vi "accelTest.vi"(0 "Communication in":refnum<class "Communication.lvclass">, 1 "Game":refnum<class "Game.lvclass">, 2 "id":i32, 3 "V_accel":dbl, 4 "V_deaccel":dbl, 5 "error in (no error)":errorcluster, 6 "replace active":bool, 7 "Samples":dbl, 8 "Start":bool=TRUE) -> (14 "Communication out":refnum<class "Communication.lvclass">, 15 "Replace":bool, 16 "Game out":refnum<class "Game.lvclass">, 19 "error out":errorcluster)   [LabVIEW 2021, in "Communication.lvclass"]
uses:
  Communication.lvclass
  Game_class/Game.lvclass
  Controls/RobotModel.ctl
  Utilities_class/Utilities.lvclass
  Game_class/Game.lvclass/Game.ctl
  Team_class/Team.lvclass/Team.ctl
  Robot_class/Robot.lvclass/Robot.ctl
  Object_class/Object.lvclass/Object.ctl
  Robot_class/Read est_v_tang.vi
  Robot_class/Write v_tang.vi
  Robot_class/Write v_norm.vi
  Robot_class/Write v_ang.vi
  Object_class/Read x.vi
  Object_class/Read y.vi
  <vilib>/Analysis/_algsub.llb/Real Vector Norm.vi
  Game_class/Read NavigationTeam.vi
  Team_class/Read RobotRef.vi
  Robot_class/Read id.vi
  Team_class/Write RobotRef.vi
  Game_class/Write NavigationTeam.vi
  Ally_class/Ally.lvclass
  D:/RoboIme/horie/SSL_AI/Team_class/Team.lvclass
  Robot_class/Robot.lvclass
  D:/RoboIme/horie/SSL_AI/Object_class/Object.lvclass
  <vilib>/Analysis/1siggen.llb/Ramp Pattern by Delta.vi
  <vilib>/Analysis/NI_AALBase.lvlib
  <vilib>/Analysis/NI_AALPro.lvlib
panel:
  out "Waveform Chart 2":dbl(graph)
  out "Waveform Chart":dbl(graph)
  out "Array":T1[](array[typedef])
  out "Robot Model":T1[](array[typedef])
  in  "Test Cluster":T1
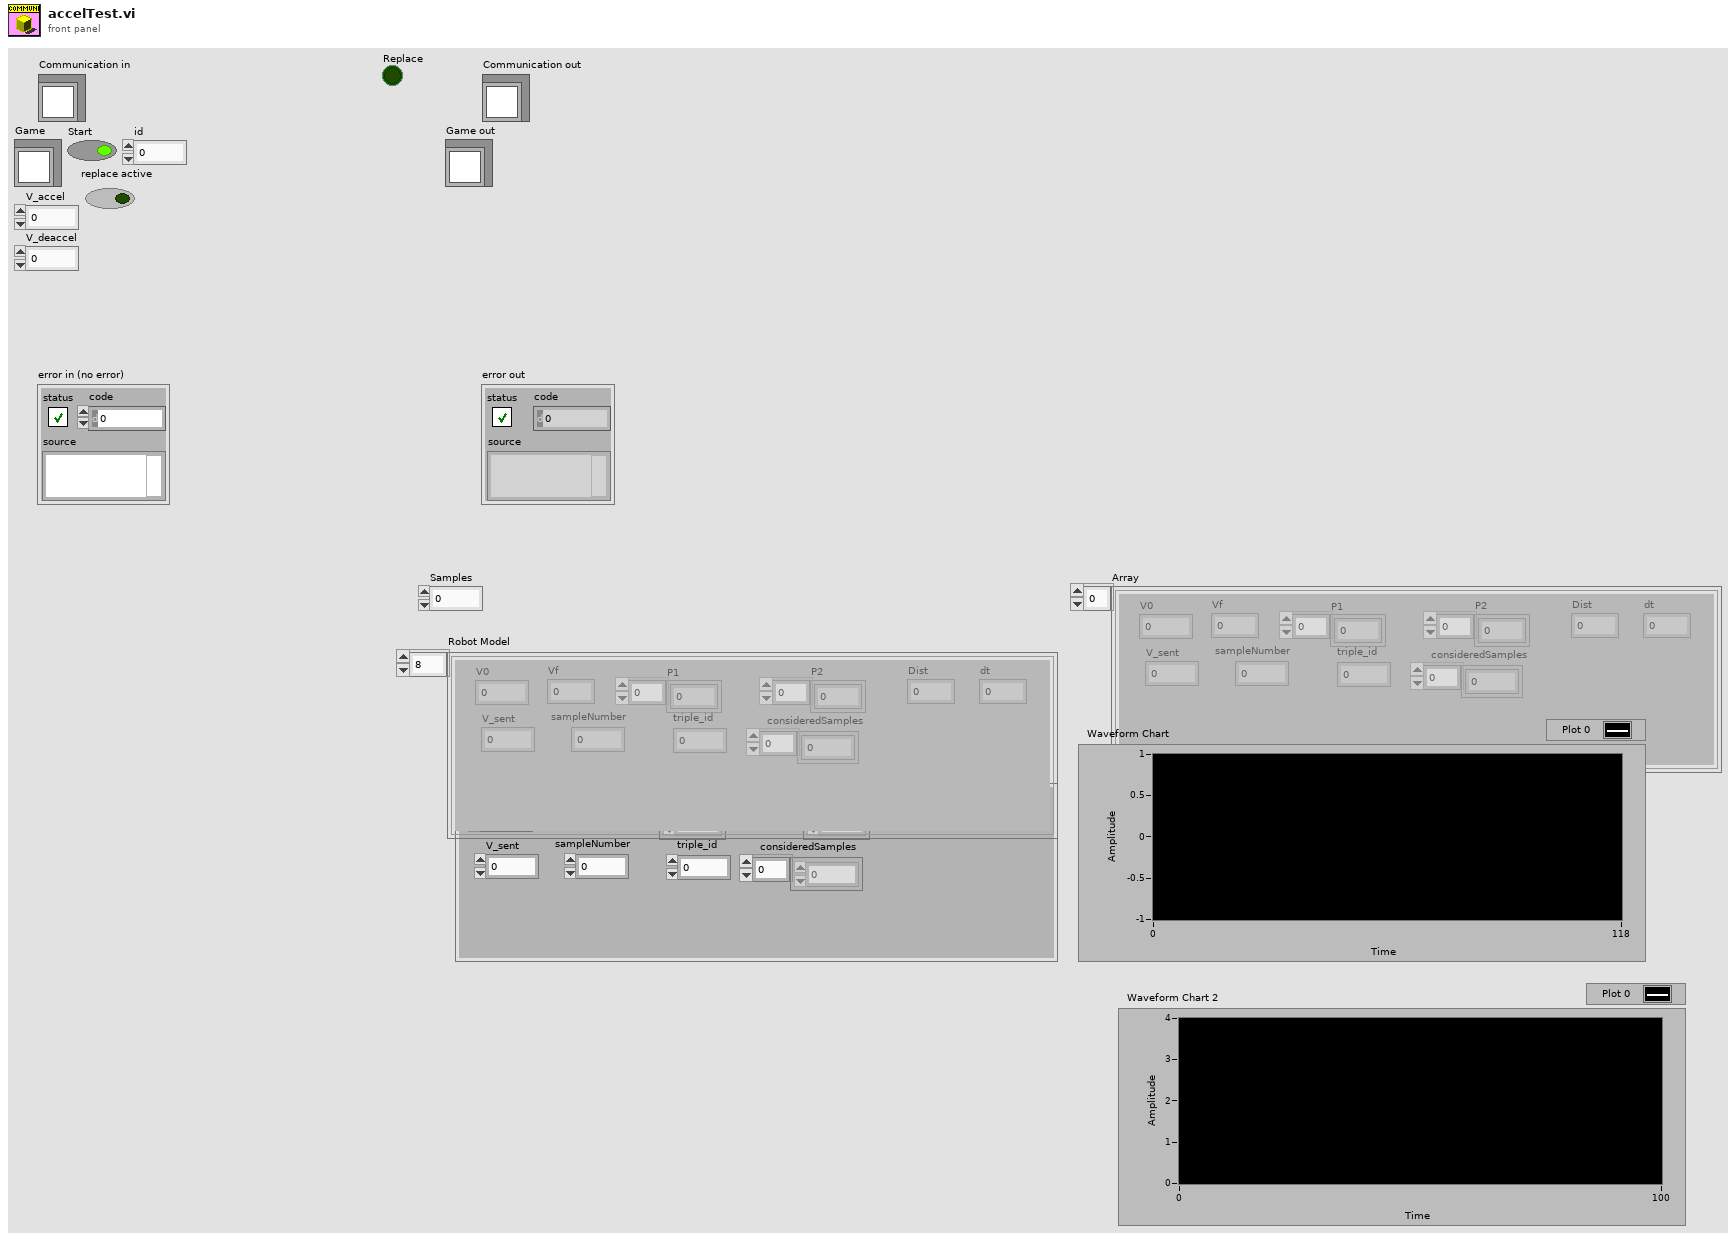
[diagram p1: front panel]
types:
  T1 = typedef "RobotModel.ctl" = cluster{"V0":dbl, "Vf":dbl, "Dist":dbl, "dt":dbl, "P1":dbl[], "P2":dbl[], "V_sent":dbl, "sampleNumber":i32, "triple_id":i32, "consideredSamples":dbl[]}
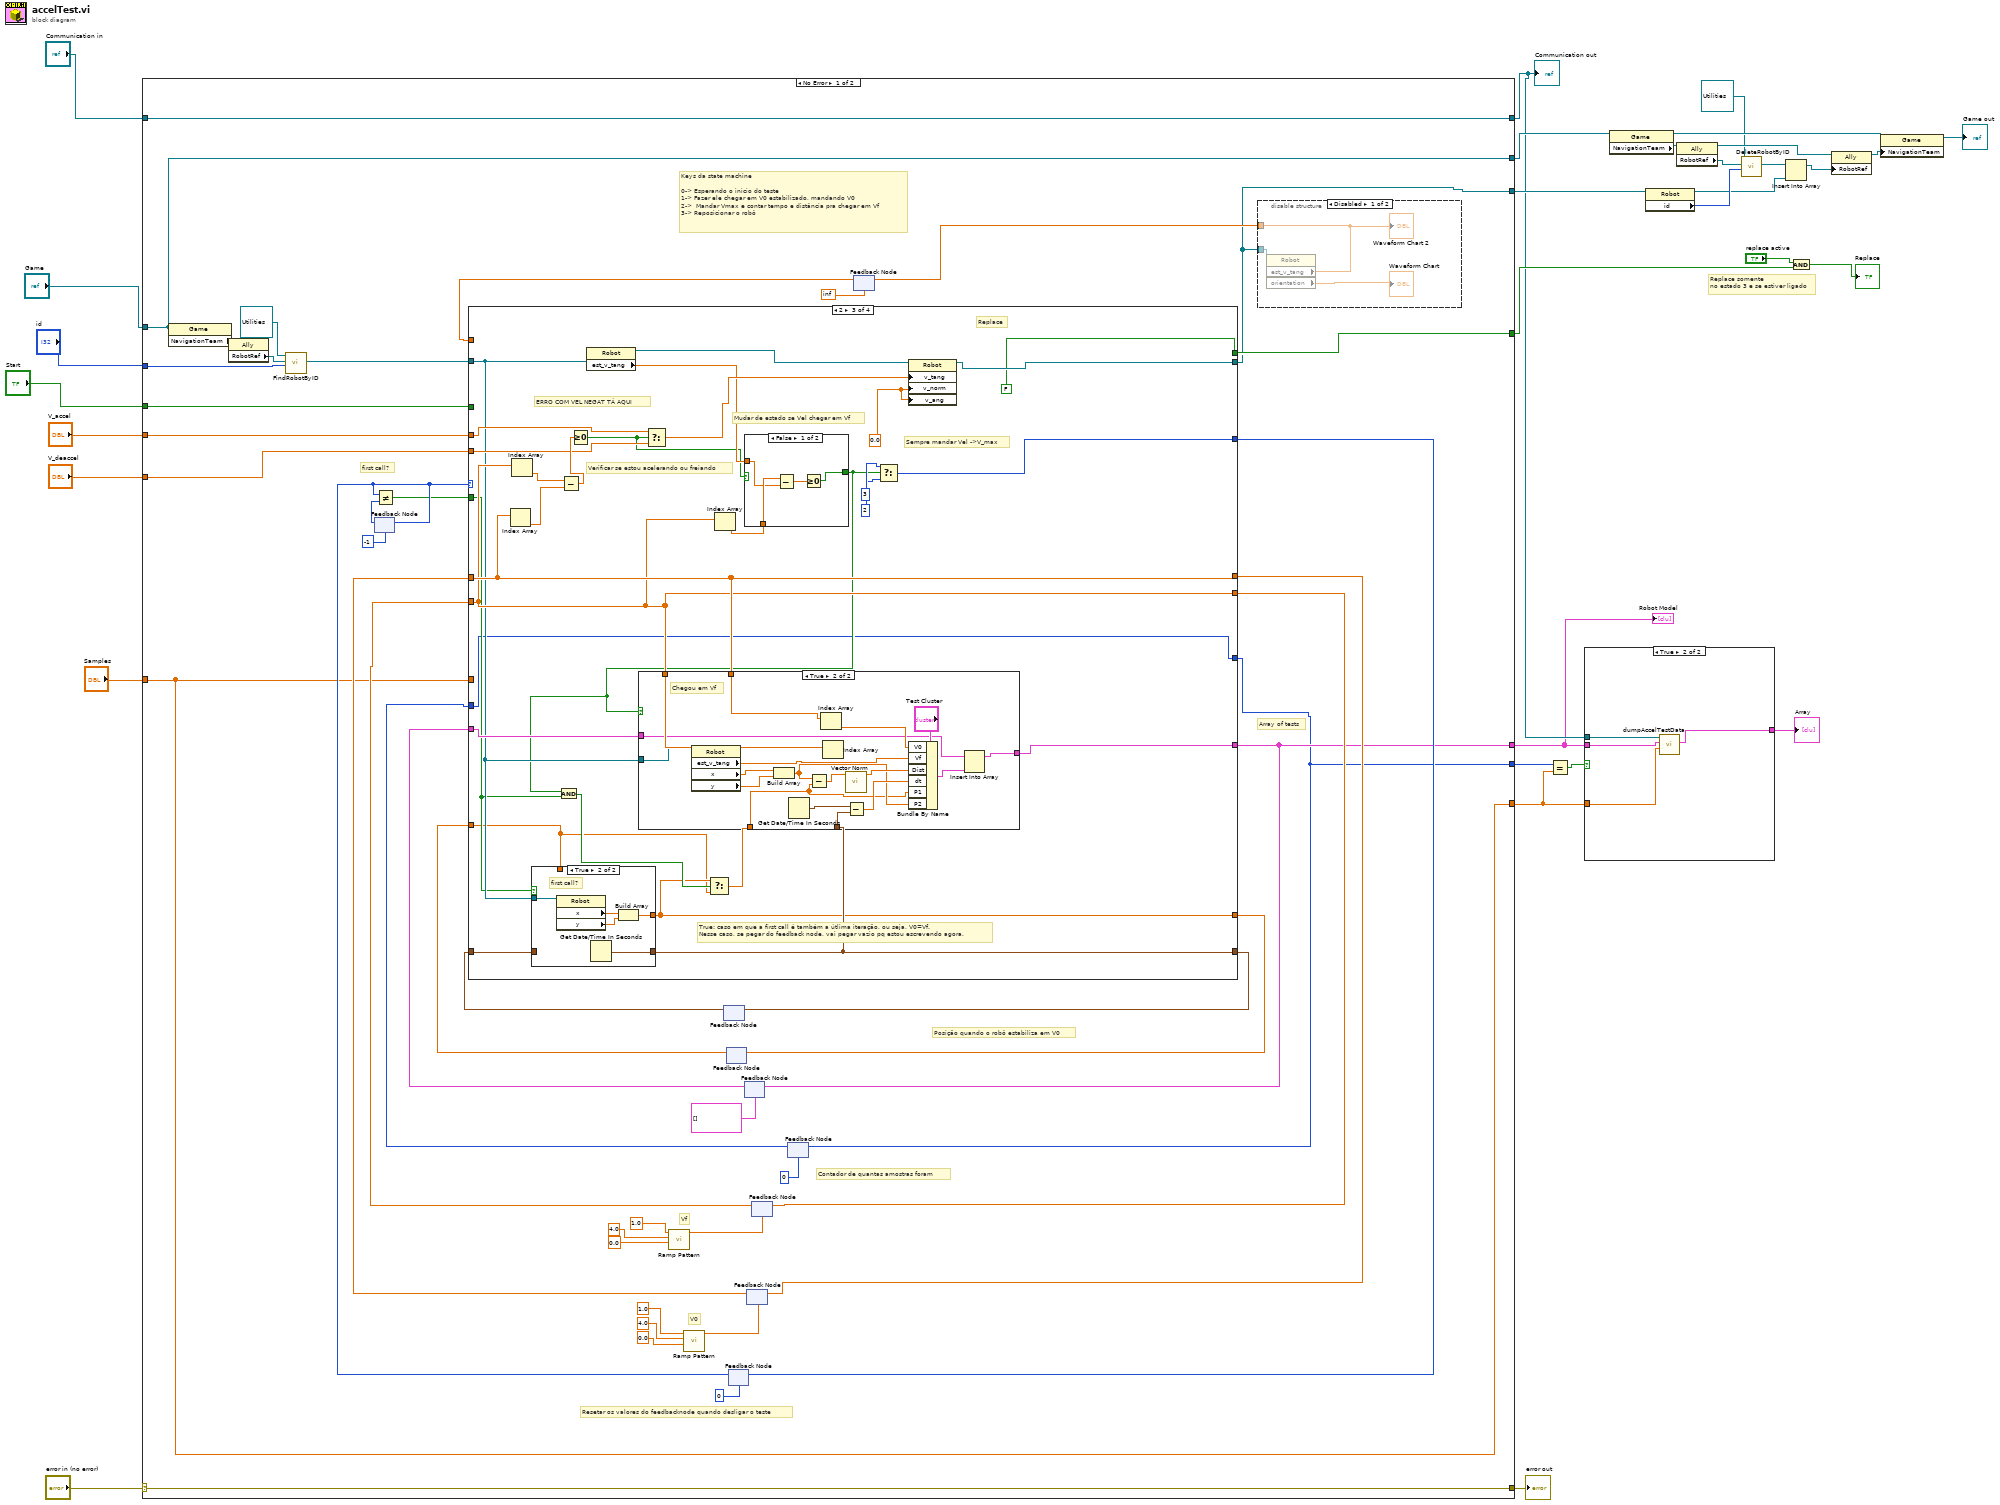
[diagram p0: block diagram]
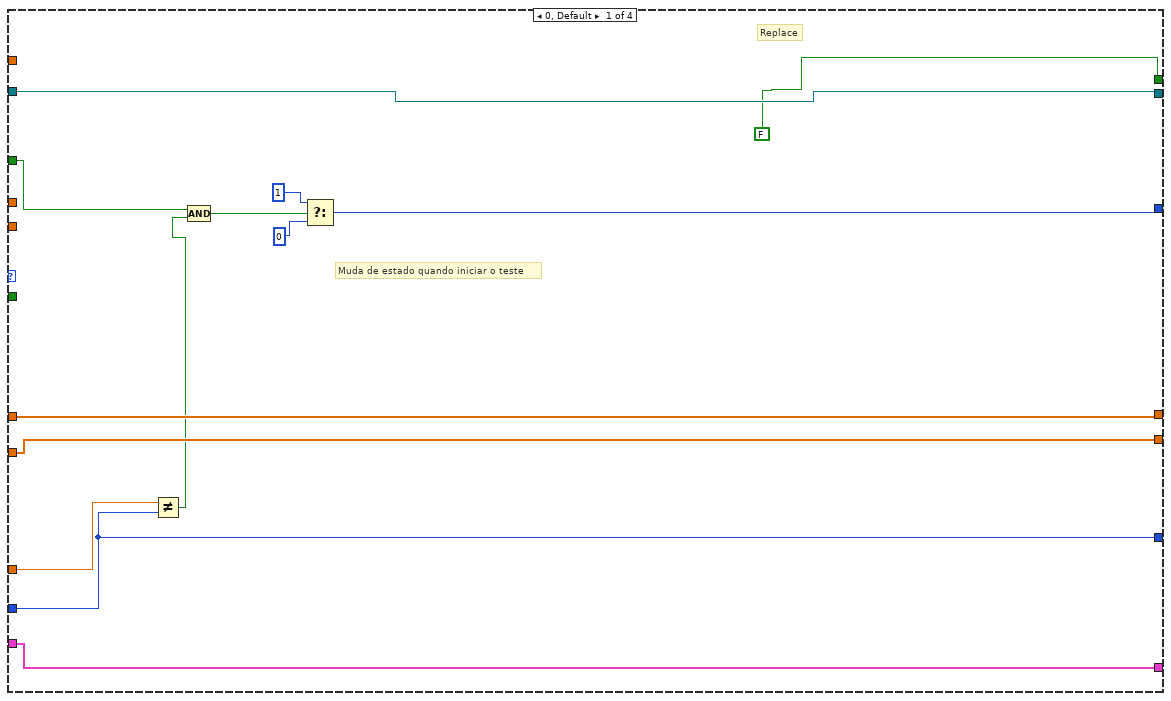
[diagram p4: hidden frame]
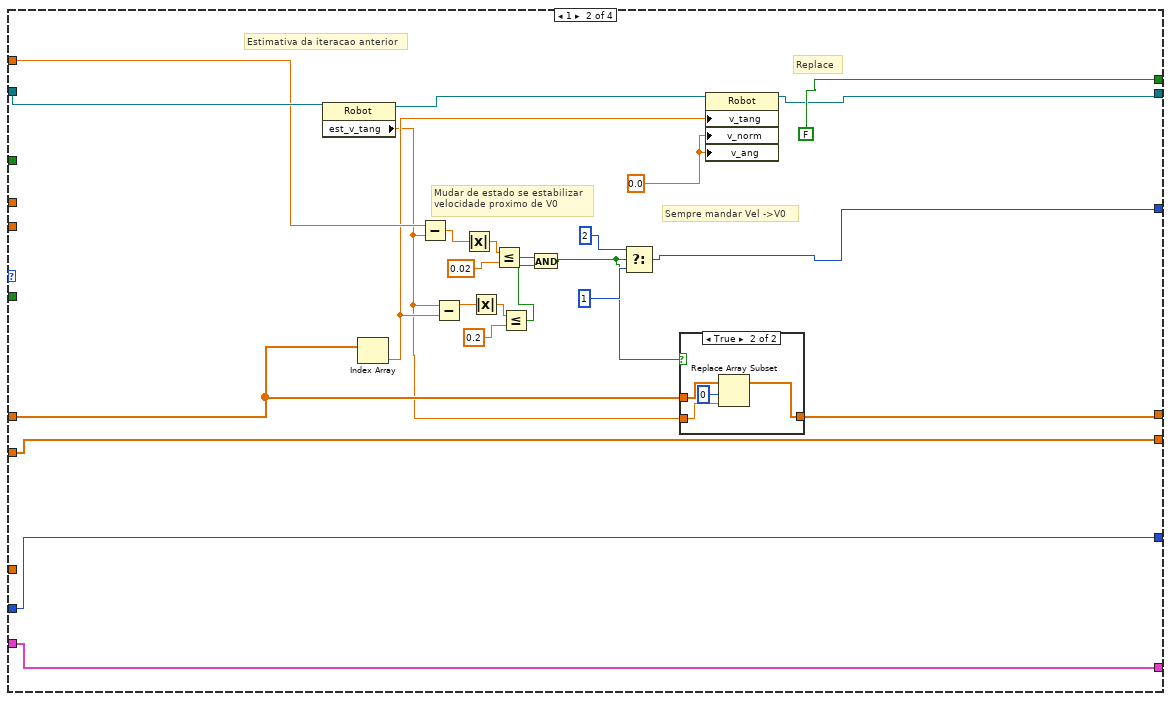
[diagram p5: hidden frame]
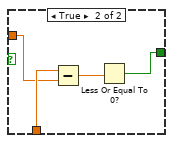
[diagram p7: hidden frame]
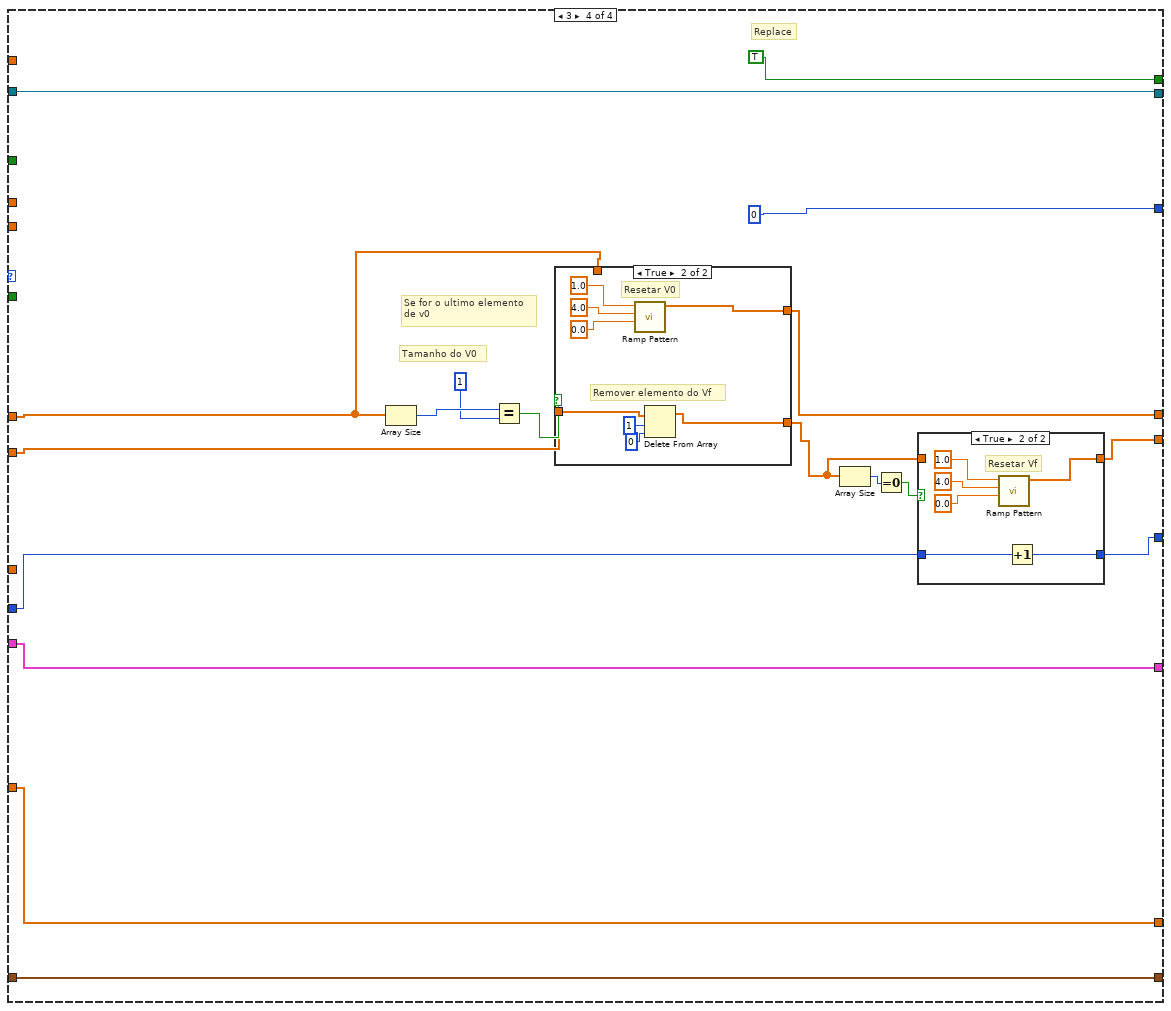
[diagram p10: hidden frame]
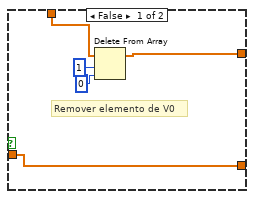
[diagram p12: hidden frame]
diagram:
  # "Replace somente\nno estado 3 e se estiver ligado"
  n1 = case shown="No Error" "error in (no error)" {
    selector: "error in (no error)" -> [w75 w227]
    tunnel: [w75 w227] -> w30
    tunnel: [w76 w226] -> w6
    tunnel: "Communication in" -> [w76 w226]
    tunnel: "Start" -> [w45 _]
    tunnel: "Game" -> [w51 _]
    tunnel: "id" -> [w70 _]
    tunnel: "V_accel" -> [w67 _]
    tunnel: "V_deaccel" -> [w66 _]
    tunnel: [w55 _] -> w23
    tunnel: [w52 _] -> w5
    tunnel: [w51 _] -> w20
    tunnel: [w32 _] -> w17
    tunnel: "Samples" -> [w35 _]
    tunnel: [w35 _] -> w4
    tunnel: [w34 _] -> w3
    frame No Error {
      # "Contador de quantas amostras foram"
      # "Posição quando o robô estabiliza em V0"
      # "Array of tests"
      # "first call?"
      # "Resetar os valores do feedbacknode quando desligar o teste"
      # "Vf"
      # "V0"
      # "Keys da state machine\n\n0-> Esperando o inicio do teste\n1-> Fazer ele chegar em V0 estabilizado, mandando V0\n2->  Mandar Vmax e contar tempo e distância pra chegar em Vf \n3-> Reposicionar o robô"
      n2 = property class="Game"(reference=w51) -> ("NavigationTeam"=w72:refnum<class "Ally.lvclass">)  [unwired: 1 in, 2 out]
      n3 = property class="Ally"(reference=w72) -> ("RobotRef"=w71:refnum<class "Robot.lvclass">[])  [unwired: 1 in, 2 out]
      n4 = call "FindRobotByID.vi"("id"=w70, "RobotRef"=w71, "Utilities in"=refnum<class "Utilities.lvclass"> refnum) -> ("Robot"=w68:refnum<class "Robot.lvclass">)  [unwired: 5 in, 3 out]
      n5 = feedback #1(-1) -> (w44:i32)
      n6 = call-poly <vilib>:"Ramp Pattern.vi"("start"=0.0, "end"=4.0, "delta"=1.0) -> ("Ramp Pattern"=w56:dbl[])  [unwired: 6 in, 2 out]
      n7 = call-poly <vilib>:"Ramp Pattern.vi"("start"=0.0, "end"=4.0, "delta"=1.0) -> ("Ramp Pattern"=w60:dbl[])  [unwired: 6 in, 2 out]
      n8 = feedback #2() -> (w50:timestamp)  [unwired: 1 in]
      n9 = feedback #3() -> (w49:dbl[])  [unwired: 1 in]
      n10 = feedback #4(0) -> (w41:i32)
      n11 = feedback-in #1(w41) -> ()
      n12 = Not Equal?(x=w41, y=w44) -> (x != y?=w40:bool)
      n13 = feedback #5(T1[] [] ("Array")) -> (w48:T1[])
      n14 = feedback #6(w60) -> (w46:dbl[])
      n15 = feedback #7(w56) -> (w47:dbl[])
      n16 = feedback #8(0) -> (w36:i32)
      n17 = feedback #9(inf) -> (w39:dbl)
      n18 = case shown="2" w41 {
        tunnel: w45 -> [w86 _ _ _]
        tunnel: [w90 w98 w147 0] -> w73
        tunnel: w68 -> [w88 w109 w135 w198]
        tunnel: w46 -> [w89 w97 w139 w197]
        tunnel: w47 -> [w87 w111 w138 w195]
        tunnel: w67 -> [_ _ w145 _]
        tunnel: w66 -> [_ _ w144 _]
        tunnel: [w88 w107 w152 w198] -> w32
        tunnel: [w89 w95 w139 w200] -> w64
        tunnel: [w87 w111 w138 w189] -> w65
        tunnel: [FALSE FALSE FALSE TRUE] -> w55
        tunnel: [_ _ w136 w193] -> w54
        tunnel: [_ _ w130 w196] -> w53
        tunnel: w50 -> [_ _ w140 w193]
        tunnel: w49 -> [_ _ w129 w196]
        tunnel: [w83 w108 w134 w194] -> w52
        tunnel: w48 -> [w83 w108 w137 w194]
        tunnel: w40 -> [_ _ w133 _]
        tunnel: w39 -> [_ w105 _ _]
        tunnel: w35 -> [w81 _ _ _]
        tunnel: [w82 w93 w125 w188] -> w34
        tunnel: w36 -> [w82 w93 w125 w187]
        frame 0, Default {
          # "Replace"
          # "Muda de estado quando iniciar o teste"
          n19 = Not Equal?(x=w81, y=w82) -> (x != y?=w80:bool)
          n20 = Compound Arithmetic op=AND(w86, w80) -> (w85:bool)
          n21 = Select(t=1, s=w85, f=0) -> (s? t:f=w90:i32)
        }
        frame 1 {
          w117 = 0.0 ("v_norm")
          # "Estimativa da iteracao anterior"
          # "Replace"
          # "Mudar de estado se estabilizar\nvelocidade proximo de V0"
          # "Sempre mandar Vel ->V0"
          n22 = property class="Robot"(reference=w109) -> (reference out=w116:refnum<class "Robot.lvclass">, "est_v_tang"=w94:dbl)  [unwired: 1 in, 1 out]
          n23 = Index Array(array=w97) -> (element=w101:dbl)  [unwired: 1 in]
          n24 = Subtract(x=w105, y=w94) -> (x-y=w106:dbl)
          n25 = Subtract(x=w94, y=w101) -> (x-y=w104:dbl)
          n26 = Absolute Value(x=w106) -> (abs(x)=w115:dbl)
          n27 = Absolute Value(x=w104) -> (abs(x)=w102:dbl)
          n28 = Less Or Equal?(x=w115, y=0.02) -> (x <= y?=w100:bool)
          n29 = Less Or Equal?(x=w102, y=0.2) -> (x <= y?=w99:bool)
          n30 = And(x=w100, y=w99) -> (x .and. y?=w96:bool)
          n31 = Select(t=2, s=w96, f=1) -> (s? t:f=w98:i32)
          n32 = case shown="True" w96 {
            tunnel: w97 -> [w118 w122]
            tunnel: [w118 w119] -> w95
            tunnel: w94 -> [_ w121]
            frame False {
            }
            frame True {
              n33 = Replace Array Subset(array=w122, new element=w121, index=0) -> (w119:dbl[])
            }
          }
          n34 = property class="Robot"(reference=w116, "v_tang"=w101, "v_norm"=w117, "v_ang"=w117) -> (reference out=w107:refnum<class "Robot.lvclass">)  [unwired: 1 in, 1 out]
        }
        frame 2 {
          w151 = 0.0 ("v_norm")
          # "ERRO COM VEL NEGAT TÁ AQUI"
          # "True: caso em que a first call é também a útlima iteração, ou seja, V0=Vf.\nNesse caso, se pegar do feedback node, vai pegar vazio pq estou escrevendo agora."
          # "Replace"
          # "Verificar se estou acelerando ou freiando"
          # "Mudar de estado se Vel chegar em Vf"
          # "Sempre mandar Vel ->V_max"
          n35 = Index Array(array=w139) -> (element=w123:dbl)  [unwired: 1 in]
          n36 = Index Array(array=w138) -> (element=w124:dbl)  [unwired: 1 in]
          n37 = case shown="True" w133 {
            tunnel: [w181 w186] -> w136
            tunnel: w140 -> [w181 _]
            tunnel: w135 -> [_ w185]
            tunnel: [w180 w182] -> w130
            tunnel: w129 -> [w180 _]
            frame False {
            }
            frame True {
              # "first call?"
              n38 = property class="Robot"(reference=w185) -> ("x"=w184:dbl, "y"=w183:dbl)  [unwired: 1 in, 2 out]
              n39 = Get Date/Time In Seconds() -> (seconds since 1Jan1904=w186:timestamp)
              n40 = Build Array(w184, w183) -> (w182:dbl[])
            }
          }
          n41 = Subtract(x=w124, y=w123) -> (x-y=w146:dbl)
          n42 = Greater Or Equal To 0?(x=w146) -> (x >= 0?=w126:bool)
          n43 = property class="Robot"(reference=w135) -> (reference out=w150:refnum<class "Robot.lvclass">, "est_v_tang"=w127:dbl)  [unwired: 1 in, 1 out]
          n44 = Select(t=w145, s=w126, f=w144) -> (s? t:f=w143:dbl)
          n45 = Index Array(array=w138) -> (element=w141:dbl)  [unwired: 1 in]
          n46 = case shown="False" w126 {
            tunnel: w141 -> [w156 w160]
            tunnel: [w153 w157] -> w132
            tunnel: w127 -> [w155 w159]
            frame False {
              n47 = Subtract(x=w156, y=w155) -> (x-y=w154:dbl)
              n48 = Greater Or Equal To 0?(x=w154) -> (x >= 0?=w153:bool)
            }
            frame True {
              n49 = Subtract(x=w160, y=w159) -> (x-y=w158:dbl)
              n50 = Less Or Equal To 0?(x=w158) -> (x <= 0?=w157:bool)
            }
          }
          n51 = And(x=w132, y=w133) -> (x .and. y?=w131:bool)
          n52 = Select(t=w130, s=w131, f=w129) -> (s? t:f=w128:dbl[])
          n53 = case shown="True" w132 {
            tunnel: w139 -> [_ w173]
            tunnel: w138 -> [_ w172]
            tunnel: w135 -> [_ w171]
            tunnel: w137 -> [w161 w166]
            tunnel: [w161 w164] -> w134
            tunnel: w136 -> [_ w169]
            tunnel: w128 -> [_ w163]
            frame False {
            }
            frame True {
              # "Chegou em Vf"
              n54 = property class="Robot"(reference=w171) -> ("est_v_tang"=w162:dbl, "x"=w179:dbl, "y"=w178:dbl)  [unwired: 1 in, 2 out]
              n55 = Build Array(w179, w178) -> (w167:dbl[])
              n56 = Get Date/Time In Seconds() -> (seconds since 1Jan1904=w170:timestamp)
              n57 = Subtract(x=w167, y=w163) -> (x-y=w176:dbl[])
              n58 = Index Array(array=w173) -> (element=w174:dbl)  [unwired: 1 in]
              n59 = Index Array(array=w172) -> ()  [unwired: 1 in, 1 out]
              n60 = call-poly <vilib>:"Vector Norm.vi"("Input Vector"=w176) -> ("norm"=w175:dbl)  [unwired: 9 in, 1 out]
              n61 = Subtract(x=w170, y=w169) -> (x-y=w168:dbl)
              n62 = Bundle By Name(cluster="Test Cluster", "V0"=w174, "Vf"=w162, "Dist"=w175, "dt"=w168, "P1"=w163, "P2"=w167) -> (w165:T1)
              n63 = Insert Into Array(array=w166, new element=w165) -> (w164:T1[])  [unwired: 1 in]
            }
          }
          n64 = Select(t=3, s=w132, f=2) -> (s? t:f=w147:i32)
          n65 = property class="Robot"(reference=w150, "v_tang"=w143, "v_norm"=w151, "v_ang"=w151) -> (reference out=w152:refnum<class "Robot.lvclass">)  [unwired: 1 in, 1 out]
        }
        frame 3 {
          # "Se for o ultimo elemento\nde v0"
          # "Replace"
          # "Tamanho do V0"
          n66 = Array Size(array=w197) -> (size(s)=w203:i32)
          n67 = Equal?(x=w203, y=1) -> (x = y?=w201:bool)
          n68 = case shown="True" w201 {
            tunnel: [w214 w222] -> w200
            tunnel: w197 -> [w217 _]
            tunnel: w195 -> [w213 w221]
            tunnel: [w213 w218] -> w190
            frame False {
              # "Remover elemento de V0"
              n69 = Delete From Array(array=w217, length=1, index=0) -> (array with subset deleted=w214:dbl[])  [unwired: 1 out]
            }
            frame True {
              # "Remover elemento do Vf"
              # "Resetar V0"
              n70 = call-poly <vilib>:"Ramp Pattern.vi"("start"=0.0, "end"=4.0, "delta"=1.0) -> ("Ramp Pattern"=w222:dbl[])  [unwired: 6 in, 2 out]
              n71 = Delete From Array(array=w221, length=1, index=0) -> (array with subset deleted=w218:dbl[])  [unwired: 1 out]
            }
          }
          n72 = Array Size(array=w190) -> (size(s)=w192:i32)
          n73 = Equal To 0?(x=w192) -> (x = 0?=w191:bool)
          n74 = case shown="True" w191 {
            tunnel: w190 -> [w206 _]
            tunnel: [w206 w209] -> w189
            tunnel: [w205 w208] -> w188
            tunnel: w187 -> [w205 w207]
            frame False {
            }
            frame True {
              # "Resetar Vf"
              n75 = call-poly <vilib>:"Ramp Pattern.vi"("start"=0.0, "end"=4.0, "delta"=1.0) -> ("Ramp Pattern"=w209:dbl[])  [unwired: 6 in, 2 out]
              n76 = Increment(x=w207) -> (x+1=w208:i32)
            }
          }
        }
      }
      n77 = feedback-in #2(w54) -> ()
      n78 = feedback-in #3(w53) -> ()
      n79 = feedback-in #4(w73) -> ()
      n80 = feedback-in #5(w52) -> ()
      n81 = feedback-in #6(w64) -> ()
      n82 = feedback-in #7(w65) -> ()
      n83 = feedback-in #8(w34) -> ()
      n84 = disable-structure shown="Disabled" {
        disable-tunnel: [w78 _] -> w33
        disable-tunnel: w32 -> [w77 _]
        frame Disabled {
          n85 = property class="Robot"(reference=w77) -> ("est_v_tang"=w78:dbl, "orientation"=→"Waveform Chart":dbl)  [unwired: 1 in, 2 out]
          "Waveform Chart 2" <- w78
        }
        frame Enabled {
        }
      }
      n86 = feedback-in #9(w33) -> ()
    }
    frame Error {
    }
  }
  "error out" <- w30
  "Communication out" <- w6
  "Robot Model" <- w5
  n87 = Equal?(x=w3, y=w4) -> (x = y?=w2:bool)
  n88 = case shown="True" w2 {
    tunnel: w4 -> [_ w231]
    tunnel: w6 -> [_ w230]
    tunnel: w5 -> [_ w229]
    tunnel: [_ w228] -> w1
    frame False {
    }
    frame True {
      n89 = call "dumpAccelTestData.vi"("Samples"=w231, "Robot Model Array"=w229, "Communication in"=w230) -> ("Mean"=w228:T1[])  [unwired: 6 in, 2 out]
    }
  }
  "Array" <- w1
  n90 = property class="Game"(reference=w20) -> (reference out=w11:refnum<class "Game.lvclass">, "NavigationTeam"=w19:refnum<class "Ally.lvclass">)  [unwired: 1 in, 1 out]
  n91 = property class="Robot"(reference=w17) -> (reference out=w14:refnum<class "Robot.lvclass">, "id"=w16:i32)  [unwired: 1 in, 1 out]
  n92 = property class="Ally"(reference=w19) -> (reference out=w13:refnum<class "Ally.lvclass">, "RobotRef"=w18:refnum<class "Robot.lvclass">[])  [unwired: 1 in, 1 out]
  n93 = call "DeleteRobotByID.vi"("id"=w16, "RobotRef"=w18, "Utilities in"=refnum<class "Utilities.lvclass"> refnum) -> ("RobotRef out"=w15:refnum<class "Robot.lvclass">[])  [unwired: 6 in, 2 out]
  n94 = Insert Into Array(array=w15, new element=w14) -> (w12:refnum<class "Robot.lvclass">[])  [unwired: 1 in]
  n95 = And(x="replace active", y=w23) -> (x .and. y?=→"Replace":bool)
  n96 = property class="Ally"(reference=w13, "RobotRef"=w12) -> (reference out=w10:refnum<class "Ally.lvclass">)  [unwired: 1 in, 1 out]
  n97 = property class="Game"(reference=w11, "NavigationTeam"=w10) -> (reference out=→"Game out":refnum<class "Game.lvclass">)  [unwired: 1 in, 1 out]
